vi "update Test.vi"(8 "error in (no error)":errorcluster, 10 "updated Test":refnum<class "Test.lvclass">, 11 "Norm in":refnum<class "Norm.lvclass">) -> (0 "error out":errorcluster, 3 "Norm out":refnum<class "Norm.lvclass">)   [LabVIEW 2013, in "DatenKlassen.lvlib" / "Norm.lvclass"]
uses:
  Norm.lvclass
  Test/Test.lvclass
  Norm.lvclass/Norm.ctl
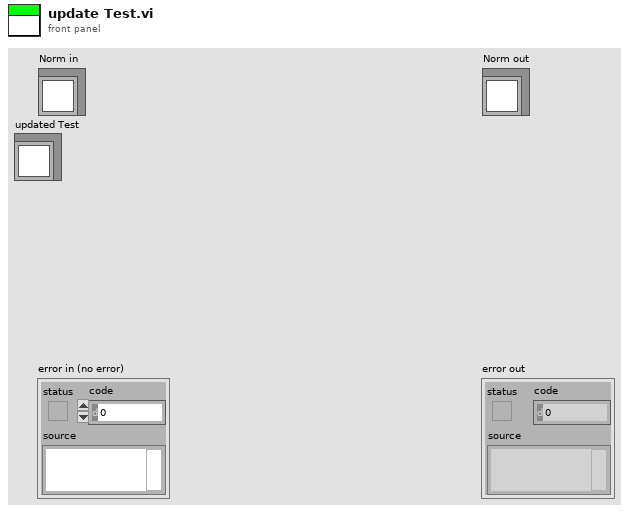
[diagram p1: front panel]
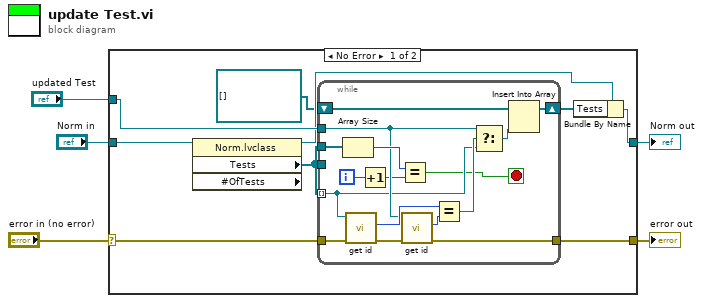
[diagram p0: block diagram]
diagram:
  n1 = case shown="No Error" "error in (no error)" {
    selector: "error in (no error)" -> [w12 w32]
    tunnel: [w11 w32] -> w4
    tunnel: [w9 w31] -> w1
    tunnel: "Norm in" -> [w14 w31]
    tunnel: "updated Test" -> [w13 _]
    frame No Error {
      n2 = property class="Norm.lvclass" props=["Tests", "#OfTests"](reference=w14) -> (reference out=w10:refnum<class "Norm.lvclass">, "Tests"=w7:refnum<class "Test.lvclass">[])  [unwired: 1 in, 2 out]
      n3 = while {
        tunnel: w7 -> [w22] mode=indexing
        tunnel: w13 -> [w23]
        tunnel: w12 -> [w28]
        tunnel: [w26] -> w11
        tunnel: w7 -> [_]
        shift-right: [w16] -> w8
        shift-left: refnum<class "Test.lvclass">[] [] ("Tests") -> [w17]
        tunnel: w7 -> [w21]
        i -> [w20]
        stop <- w15 stop-if-true
        n4 = Array Size(array=w21) -> (size(s)=w25:i32)
        n5 = call-dynamic "get id.vi"("error in (no error)"=w28, "Test in"=w22) -> ("error out"=w27:errorcluster, "id"=w30:u32)  [unwired: 7 in, 1 out]
        n6 = Increment(x=w20) -> (x+1=w19:i32)
        n7 = Equal?(x=w25, y=w19) -> (x = y?=w15:bool)
        n8 = call-dynamic "get id.vi"("error in (no error)"=w27, "Test in"=w23) -> ("error out"=w26:errorcluster, "id"=w29:u32)  [unwired: 7 in, 1 out]
        n9 = Equal?(x=w30, y=w29) -> (x = y?=w24:bool)
        n10 = Select(t=w23, s=w24, f=w22) -> (s? t:f=w18:refnum<class "Test.lvclass">)
        n11 = Insert Into Array(array=w17, new element=w18) -> (w16:refnum<class "Test.lvclass">[])  [unwired: 1 in]
      }
      n12 = Bundle By Name(cluster=w10, "Tests"=w8) -> (w9:refnum<class "Norm.lvclass">)
    }
    frame Error {
    }
  }
  "error out" <- w4
  "Norm out" <- w1
